vi "is a.vi"(8 "error in (no error)":errorcluster, 11 "GaugeController in":refnum<class "GaugeController.lvclass">) -> (0 "error out":errorcluster, 2 "is a":string, 3 "GaugeController out":refnum<class "GaugeController.lvclass">)   [LabVIEW 2016, in "Hardware.lvlib" / "GaugeController.lvlib" / "GaugeController.lvclass"]
uses:
  <userlib>/Common Components/Hardware/GaugeController/GaugeController/GaugeController.lvclass
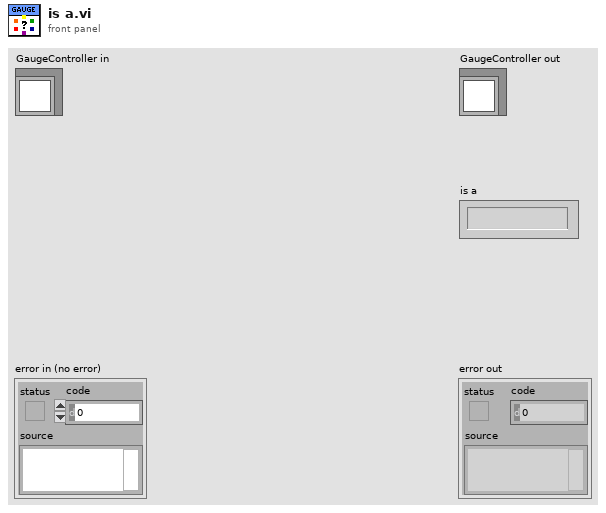
[diagram p1: front panel]
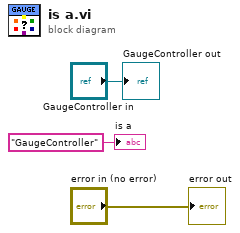
[diagram p0: block diagram]
diagram:
  "error out" <- "error in (no error)"
  "GaugeController out" <- "GaugeController in"
  "is a" <- "GaugeController" ("is a")
